vi "parse_get_all_collection_response.vi"(0 "headers":string, 5 "body":string, 11 "error in (no error)":errorcluster) -> (4 "collection_list":string[](array[string]), 15 "error out":errorcluster)   [LabVIEW 2020, in "vector_weviate.lvclass"]
uses:
  vector_weviate.lvclass
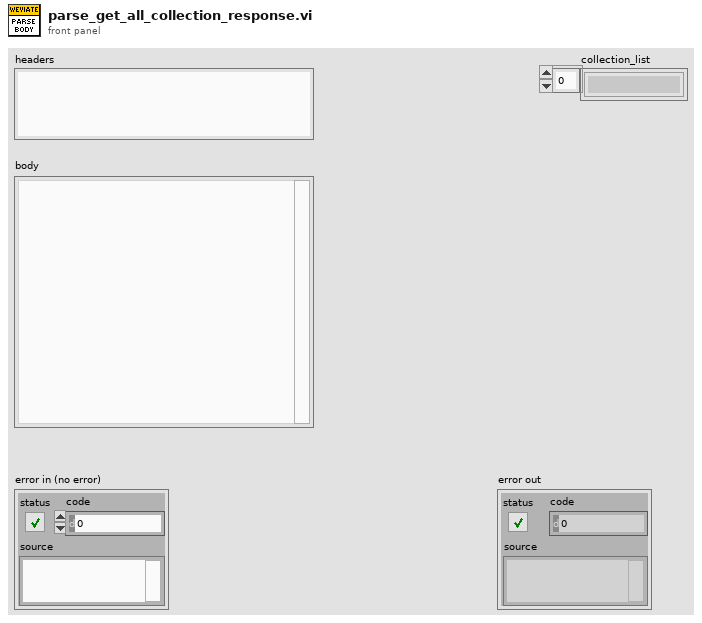
[diagram p1: front panel]
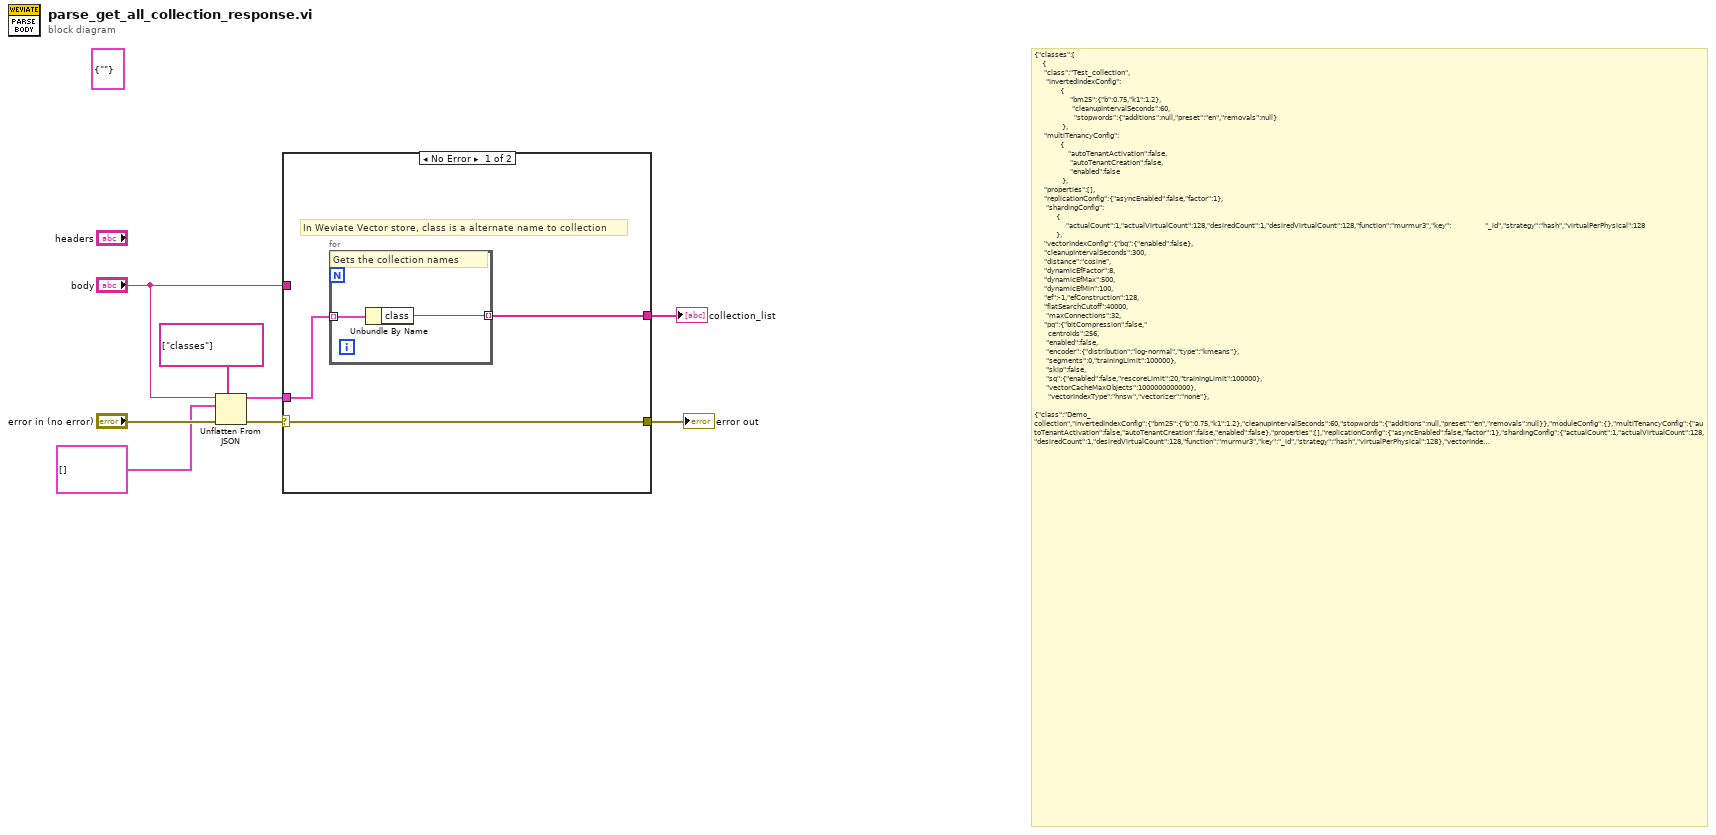
[diagram p0: block diagram]
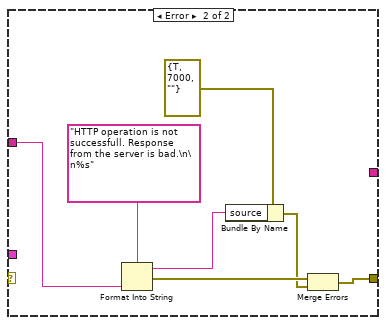
[diagram p2: hidden frame]
diagram:
  (unwired) cluster{"class":string} {"class"=""}
  # "{\"classes\":[\n    {\n     \"class\":\"Test_collection\",\n      \"invertedIndexConfig\":\n             {\n                  \"bm25\":{\"b\":0.75,\"k1\":1.2},\n                   \"cleanupIntervalSeconds\":60,\n                    \"stopwords\":{\"additions\":null,\"preset\":\"en\",\"removals\":null}\n              },\n     \"multiTenancyConfig\":\n             {\n                 \"autoTenantActivation\":false,\n                  \"autoTenantCreation\":false,\n                  \"enabled\":false\n              },\n     \"properties\":[],\n     \"replicationConfig\":{\"asyncEnabled\":false,\"factor\":1},\n      \"shardingConfig\":\n           {\n                \"actualCount\":1,\"actualVirtualCount\":128,\"desiredCount\":1,\"desiredVirtualCount\":128,\"function\":\"murmur3\",\"key\":                 \"_id\",\"strategy\":\"hash\",\"virtualPerPhysical\":128\n           },\n     \"vectorIndexConfig\":{\"bq\":{\"enabled\":false},\n     \"cleanupIntervalSeconds\":300,\n     \"distance\":\"cosine\",\n     \"dynamicEfFactor\":8,\n     \"dynamicEfMax\":500,\n     \"dynamicEfMin\":100,\n     \"ef\":-1,\"efConstruction\":128,\n     \"flatSearchCutoff\":40000,\n      \"maxConnections\":32,\n     \"pq\":{\"bitCompression\":false,\"\n       centroids\":256,\n      \"enabled\":false,\n      \"encoder\":{\"distribution\":\"log-normal\",\"type\":\"kmeans\"},\n      \"segments\":0,\"trainingLimit\":100000},\n      \"skip\":false,\n      \"sq\":{\"enabled\":false,\"rescoreLimit\":20,\"trainingLimit\":100000},\n      \"vectorCacheMaxObjects\":1000000000000},\n       \"vectorIndexType\":\"hnsw\",\"vectorizer\":\"none\"},\n\n{\"class\":\"Demo_collection\",\"invertedIndexConfig\":{\"bm25\":{\"b\":0.75,\"k1\":1.2},\"cleanupIntervalSeconds\":60,\"stopwords\":{\"additions\":null,\"preset\":\"en\",\"removals\":null}},\"moduleConfig\":{},\"multiTenancyConfig\":{\"autoTenantActivation\":false,\"autoTenantCreation\":false,\"enabled\":false},\"properties\":[],\"replicationConfig\":{\"asyncEnabled\":false,\"factor\":1},\"shardingConfig\":{\"actualCount\":1,\"actualVirtualCount\":128,\"desiredCount\":1,\"desiredVirtualCount\":128,\"function\":\"murmur3\",\"key\":\"_id\",\"strategy\":\"hash\",\"virtualPerPhysical\":128},\"vectorIndexConfig\":{\"bq\":{\"enabled\":false},\"cleanupIntervalSeconds\":300,\"distance\":\"cosine\",\"dynamicEfFactor\":8,\"dynamicEfMax\":500,\"dynamicEfMin\":100,\"ef\":-1,\"efConstruction\":128,\"flatSearchCutoff\":40000,\"maxConnections\":32,\"pq\":{\"bitCompression\":false,\"centroids\":256,\"enabled\":false,\"encoder\":{\"distribution\":\"log-normal\",\"type\":\"kmeans\"},\"segments\":0,\"trainingLimit\":100000},\"skip\":false,\"sq\":{\"enabled\":false,\"rescoreLimit\":20,\"trainingLimit\":100000},\"vectorCacheMaxObjects\":1000000000000},\"vectorIndexType\":\"hnsw\",\"vectorizer\":\"none\"}]}"
  n1 = Unflatten From JSON(path=string[] ["classes"], JSON string="body", type and defaults=cluster{"class":string}[] [], error in (no error)="error in (no error)") -> (value=w5:cluster{"class":string}[], error out=w6:errorcluster)  [unwired: 3 in]
  n2 = case shown="No Error" w6 {
    selector: w6 -> [w11 _]
    tunnel: w5 -> [w10 _]
    tunnel: [w11 w14] -> w4
    tunnel: [w9 _] -> w2
    tunnel: "body" -> [_ w17]
    frame No Error {
      # "In Weviate Vector store, class is a alternate name to collection"
      n3 = for {
        tunnel: w10 -> [w13] mode=indexing
        tunnel: [w12] -> w9 mode=indexing
        # "Gets the collection names"
        n4 = Unbundle By Name(w13) -> ("class"=w12:string)
      }
    }
    frame Error {
      n5 = Format Into String(format string="HTTP operation is not successfull. Response from the server is bad.\n\n%s", w17) -> (resulting string=w19:string, error out=w16:errorcluster)  [unwired: 2 in]
      n6 = Bundle By Name(cluster=errorcluster {"status"=TRUE, "code"=7000, "source"=""} ("error constant"), "source"=w19) -> (w15:errorcluster)
      n7 = Merge Errors(w16, w15) -> (w14:errorcluster)
    }
  }
  "error out" <- w4
  "collection_list" <- w2
